vi "Lockin.Engine.vi"(8 "error in (no error)":errorcluster, 11 "Instrument.DAQ":refnum<class "Instrument.DAQ.lvclass">) -> (0 "error out":errorcluster, 2 "<Results> (X,Y,R,Theta,Mean)":T1 {"Results (Dictionary)"."value" format="%#_6p"}, 3 "Instrument.DAQ out":refnum<class "Instrument.DAQ.lvclass">)   [LabVIEW 2019, in "DSP.lvclass"]
uses:
  DSP.lvclass
  Instrument.DAQ/Instrument.DAQ.lvclass
  Instrument.DAQ/Typedefs/Results--Cluster.ctl
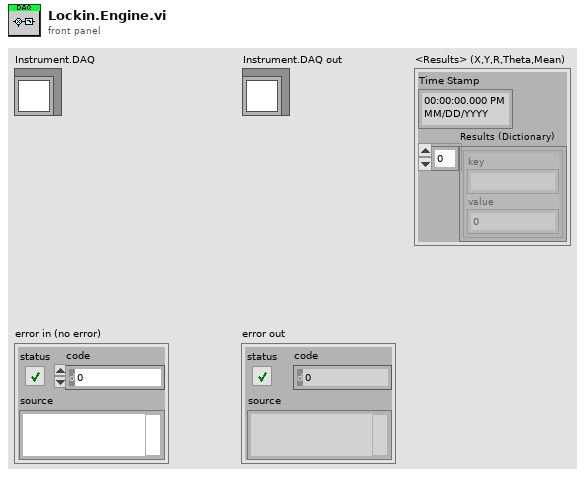
[diagram p1: front panel]
types:
  T1 = typedef "Instrument.Lockin.lvlib/Instrument.DAQ.lvclass/Results--Cluster.ctl" = cluster{"Time Stamp":timestamp, "Results (Dictionary)":cluster{"key":string, "value":dbl}[]}
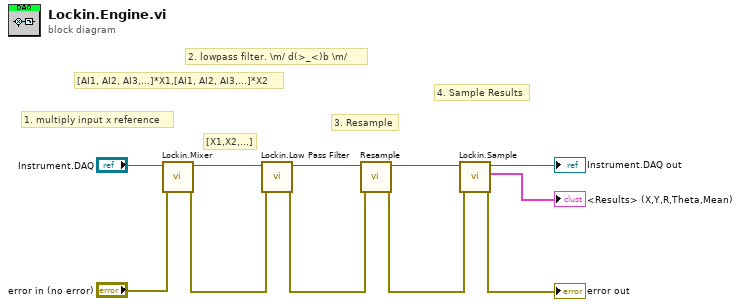
[diagram p0: block diagram]
diagram:
  # "4. Sample Results"
  # "3. Resample"
  # "[X1,X2,...]"
  # "1. multiply input x reference"
  # "2. lowpass filter. \\m/ d(>_<)b \\m/"
  # "[AI1, AI2, AI3,...]*X1,[AI1, AI2, AI3,...]*X2"
  n1 = call "Lockin.Mixer.vi"("error in (no error)"="error in (no error)", "Instrument.DAQ"="Instrument.DAQ") -> ("error out"=w9:errorcluster, "Instrument.DAQ"=w11:refnum<class "Instrument.DAQ.lvclass">)  [unwired: 8 in]
  n2 = call "Lockin.Low Pass Filter.vi"("error in (no error)"=w9, "Lockin.DAQ"=w11) -> ("error out"=w6:errorcluster, "Lockin.DAQ"=w7:refnum<class "Instrument.DAQ.lvclass">)  [unwired: 8 in]
  n3 = call "Resample.vi"("error in (no error)"=w6, "Instrument.DAQ"=w7) -> ("error out"=w2:errorcluster, "Instrument.DAQ out"=w5:refnum<class "Instrument.DAQ.lvclass">)  [unwired: 8 in]
  n4 = call "Lockin.Sample.vi"("error in (no error)"=w2, "Lockin.DAQ"=w5) -> ("error out"=→"error out":errorcluster, "Results"=→"<Results> (X,Y,R,Theta,Mean)":T1, "Lockin.DAQ out"=→"Instrument.DAQ out":refnum<class "Instrument.DAQ.lvclass">)  [unwired: 7 in]
